vi "Find VI with Focus__ogtk.vi"(8 "error in":errorcluster caption="error in (no error)", 9 "Exclude Callers":bool=TRUE caption="Exclude All Callers (T)", 10 "Exclude Levels":i32=-1 caption="Exclude Levels (call chain=-1)", 11 "Exclude Names":string[](array[string]) caption="Exclude Names (none)") -> (0 "error out":errorcluster, 1 "Changed?":bool, 2 "VI with Focus":refnum<vi>, 3 "Valid?":bool, 5 "VI Name":string)   [LabVIEW 2017]
doc: "Returns a reference to the frontmost VI panel. \n\nThis VI is reentrant (as indicated by the crosshatched background) so that references in use by one caller aren't closed by another. This also allows different callers to exclude different panels from consideration and to get a proper indication of whether a changed has occurred since their own last last call.\n\nThis is an enhancement of Jim Kring's Find Frontmost VI that returns a reference as well as a name, signals if this has changed since the last call, allows exclusion of VIs in the calling sequence of this VI or other VIs of the user's choice (useful for editing utilities that stay on top of all other windows), cleans up unused references, and runs, on average, 50 or more times faster.\n\nGenerates no errors.\n\nCopyright © 2003 by Paul F. Sullivan. All rights reserved. You are only permitted the usage indicated in your license agreement."
uses:
  <userlib>/_OpenG.lib/appcontrol/appcontrol.llb/Find Focus State__ogtk.ctl
panel:
  out "State Data":T2={"State"=enum."Excluded?", "Recent VI"=refnum, "Recent Number"=0, "Recent VI Name"="", "VI with Focus"=refnum, "Focus Number"=0, "Focus VI Name"="", "Valid?"=FALSE, "Changed?"=FALSE} {"Focus Number" format="%.0x"; "Recent Number" format="%.0x"}
  in  "State Data":T2={"State"=enum."Recent?", "Recent VI"=refnum, "Recent Number"=0, "Recent VI Name"="", "VI with Focus"=refnum, "Focus Number"=0, "Focus VI Name"="", "Valid?"=FALSE, "Changed?"=FALSE} {"Focus Number" format="%.0x"; "Recent Number" format="%.0x"}
  # "Find VI with Focus.vi\n\nReturns a reference to the frontmost VI panel.\n\nPlease visit http://www.OpenG.org to learn about the\nOpen Source LabVIEW software movement.\n\nNOTICE -- YOU MUST LEAVE THIS NOTICE IN PLACE.  PER THE TERMS OF THE LICENSE BELOW, YOU MAY SUBLICENSE THIS SOFTWARE \nIN ANY WAY THAT DOES NOT CONFLICT WITH THIS LICENSE.\n\n### BSD License (http://www.opensource.org/licenses/bsd-license.php) Begin ###\n \nCopyright (c) 2003, Paul F. Sullivan <Paul@SULLutions.com>\n\nAll rights reserved.\n\nRedistribution and use in source and binary forms, with or without modification, are permitted provided that the following conditions are met:\n\n    * Redistributions of source code must retain the above copyright notice, this list of conditions and the following disclaimer.\n    * Redistributions in binary form must reproduce the above copyright notice, this list of conditions and the following disclaimer in the \n       documentation and/or other materials provided with the distribution.\n    * Neither the name of SciWare, James Kring, Inc., nor the names of its contributors may be used to endorse or promote products derived \n       from this software without specific prior written permission.\n\nTHIS SOFTWARE IS PROVIDED BY THE COPYRIGHT HOLDERS AND CONTRIBUTORS \"AS IS\" AND ANY EXPRESS OR IMPLIED WARRANTIES, \nINCLUDING, BUT NOT LIMITED TO, THE IMPLIED WARRANTIES OF MERCHANTABILITY AND FITNESS FOR A PARTICULAR PURPOSE ARE \nDISCLAIMED. IN NO EVENT SHALL THE COPYRIGHT OWNER OR CONTRIBUTORS BE LIABLE FOR ANY DIRECT, INDIRECT, INCIDENTAL,\n SPECIAL, EXEMPLARY, OR CONSEQUENTIAL DAMAGES (INCLUDING, BUT NOT LIMITED TO, PROCUREMENT OF SUBSTITUTE GOODS OR \nSERVICES; LOSS OF USE, DATA, OR PROFITS; OR BUSINESS INTERRUPTION) HOWEVER CAUSED AND ON ANY THEORY OF LIABILITY, \nWHETHER IN CONTRACT, STRICT LIABILITY, OR TORT (INCLUDING NEGLIGENCE OR OTHERWISE) ARISING IN ANY WAY OUT OF THE USE \nOF THIS SOFTWARE, EVEN IF ADVISED OF THE POSSIBILITY OF SUCH DAMAGE.\n\n### BSD License End ###"
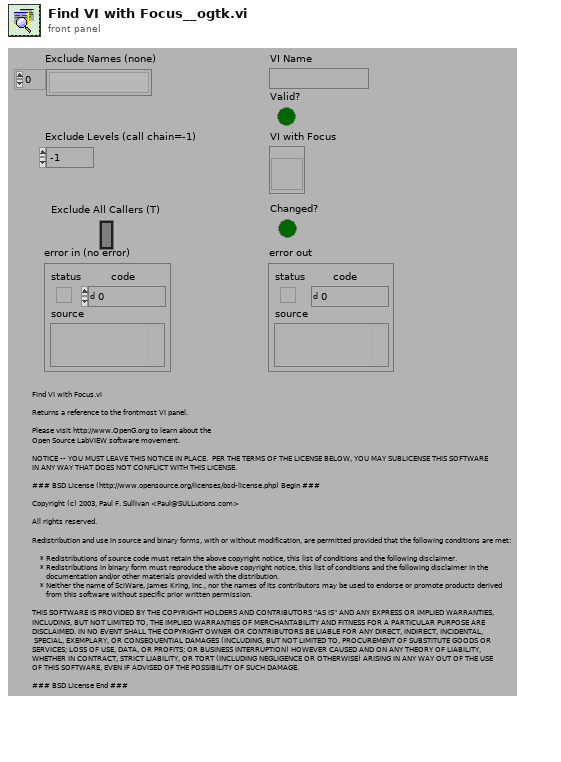
[diagram p1: front panel]
types:
  T1 = typedef "Find Focus State__ogtk.ctl" = enum16{"Initialize", "Recent?", "Accepted?", "Excluded?", "VI Panel?", "Valid?", "Done"}
  T2 = cluster{"State":T1, "Recent VI":refnum<vi>, "Recent Number":u32, "Recent VI Name":string, "VI with Focus":refnum<vi>, "Focus Number":u32, "Focus VI Name":string, "Valid?":bool, "Changed?":bool}
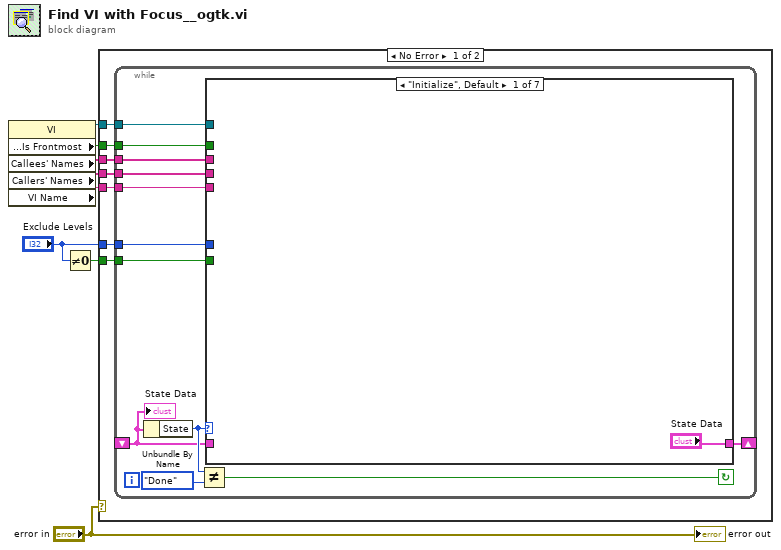
[diagram p0: block diagram]
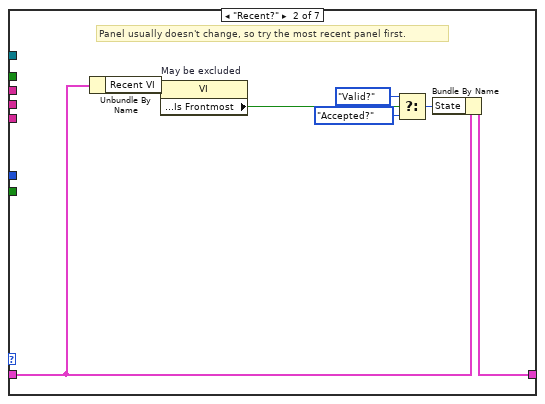
[diagram p2: hidden frame]
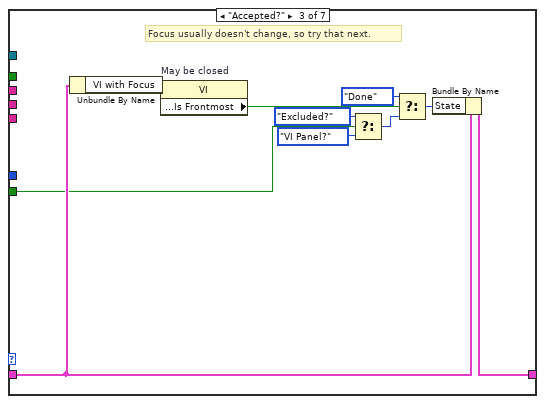
[diagram p3: hidden frame]
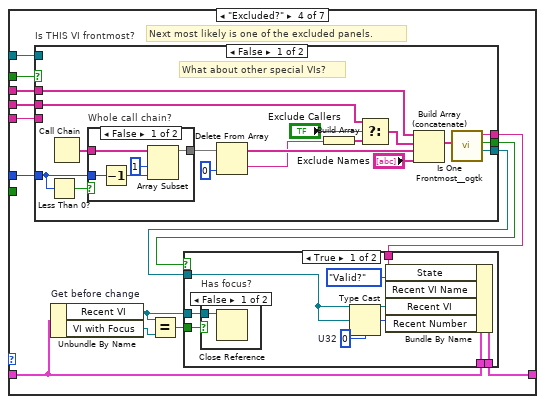
[diagram p4: hidden frame]
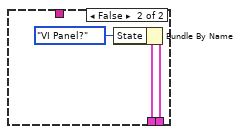
[diagram p6: hidden frame]
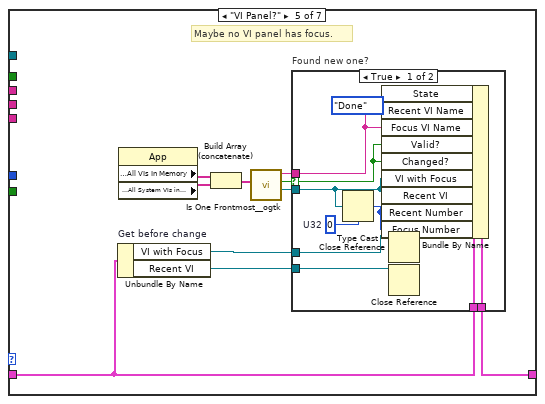
[diagram p9: hidden frame]
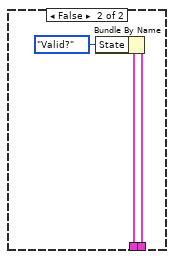
[diagram p10: hidden frame]
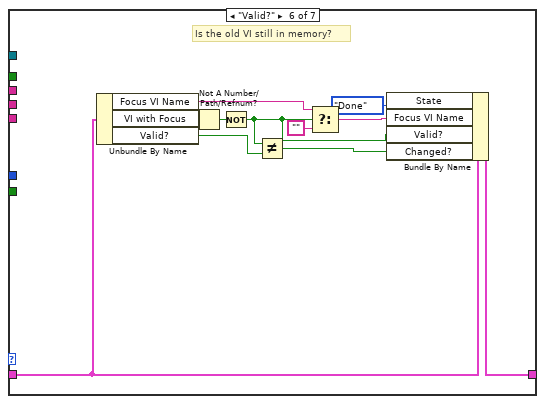
[diagram p11: hidden frame]
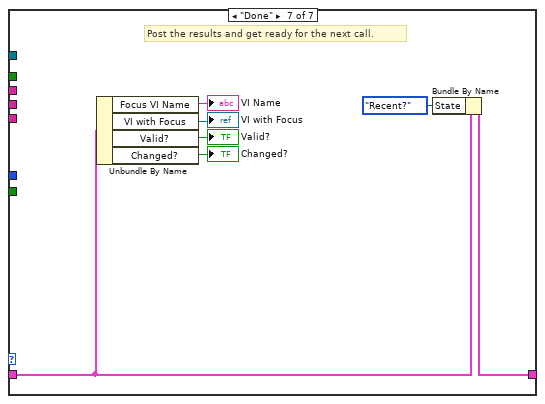
[diagram p12: hidden frame]
diagram:
  n1 = property class="VI"() -> (reference out=w4:refnum<vi>, "Front Panel Window:Is Frontmost"=w5:bool, "Callees' Names"=w7:string[], "Callers' Names"=w6:string[], "VI Name"=w1:string)  [unwired: 2 in, 1 out]
  n2 = Not Equal To 0?(x="Exclude Levels") -> (x != 0?=w2:bool)
  n3 = case shown="No Error" "error in" {
    tunnel: w6 -> [w15 _]
    tunnel: w7 -> [w14 _]
    tunnel: w5 -> [w13 _]
    tunnel: w4 -> [w12 _]
    tunnel: "Exclude Levels" -> [w11 _]
    tunnel: w2 -> [w10 _]
    tunnel: w1 -> [w9 _]
    frame No Error {
      n4 = while {
        tunnel: w9 -> [w17]
        tunnel: w10 -> [w19]
        tunnel: w11 -> [w20]
        tunnel: w12 -> [w18]
        tunnel: w13 -> [w21]
        tunnel: w14 -> [w22]
        tunnel: w15 -> [w23]
        shift-left: _ -> [w16]
        shift-right: [w25] -> _
        stop <- w24 continue-if-true
        n5 = Unbundle By Name(w16) -> ("State"=w26:T1)
        n6 = Not Equal?(x=w26, y=Find_Focus_State__ogtk."Done" ("State")) -> (x != y?=w24:bool)
        n7 = case shown="\"Initialize\", Default" w26 {
          tunnel: w21 -> [_ _ _ w59 _ _ _]
          tunnel: w23 -> [_ _ _ w58 _ _ _]
          tunnel: w22 -> [_ _ _ w57 _ _ _]
          tunnel: w20 -> [_ _ _ w56 _ _ _]
          tunnel: w19 -> [_ _ w37 _ _ _ _]
          tunnel: w16 -> [_ w34 w44 w49 w99 w129 w136]
          tunnel: ["State Data" w33 w43 w55 w104 w128 w135] -> w25
          tunnel: w18 -> [_ _ _ w52 _ _ _]
          tunnel: w17 -> [_ _ _ w50 _ _ _]
          frame "Initialize", Default {
          }
          frame "Recent?" {
            # "Panel usually doesn't change, so try the most recent panel first."
            n8 = Unbundle By Name(w34) -> ("Recent VI"=w35:refnum<vi>)
            n9 = property on="May be excluded" class="VI"(reference=w35) -> ("Front Panel Window:Is Frontmost"=w31:bool)  [unwired: 1 in, 2 out]
            n10 = Select(t=Find_Focus_State__ogtk."Valid?" ("State"), s=w31, f=Find_Focus_State__ogtk."Accepted?" ("State")) -> (s? t:f=w32:T1)
            n11 = Bundle By Name(cluster=w34, "State"=w32) -> (w33:T2)
          }
          frame "Accepted?" {
            # "Focus usually doesn't change, so try that next."
            n12 = Unbundle By Name(w44) -> ("VI with Focus"=w45:refnum<vi>)
            n13 = property on="May be closed" class="VI"(reference=w45) -> ("Front Panel Window:Is Frontmost"=w41:bool)  [unwired: 1 in, 2 out]
            n14 = Select(t=Find_Focus_State__ogtk."Excluded?" ("State"), s=w37, f=Find_Focus_State__ogtk."VI Panel?" ("State")) -> (s? t:f=w38:T1)
            n15 = Select(t=Find_Focus_State__ogtk."Done" ("State"), s=w41, f=w38) -> (s? t:f=w42:T1)
            n16 = Bundle By Name(cluster=w44, "State"=w42) -> (w43:T2)
          }
          frame "Excluded?" {
            # "Next most likely is one of the excluded panels."
            n17 = case "Is THIS VI frontmost?" shown="False" w59 {
              selector: w59 -> [_ w98]
              tunnel: w56 -> [w76 _]
              tunnel: [w75 w98] -> w54
              tunnel: w58 -> [w85 _]
              tunnel: w57 -> [w80 _]
              tunnel: [w74 w97] -> w53
              tunnel: w52 -> [_ w97]
              tunnel: [w73 w96] -> w51
              tunnel: w50 -> [_ w96]
              frame False {
                # "What about other special VIs?"
                n18 = Less Than 0?(x=w76) -> (x < 0?=w87:bool)
                n19 = Call Chain() -> (call chain=w88:string[])
                n20 = case "Whole call chain?" shown="False" w87 {
                  tunnel: w76 -> [w94 _]
                  tunnel: [w91 w95] -> w84
                  tunnel: w88 -> [w90 w95]
                  frame False {
                    n21 = Decrement(x=w94) -> (x-1=w92:i32)
                    n22 = Array Subset(array=w90, index=1 ("Array Index"), length=w92) -> (w91:string[])
                  }
                  frame True {
                  }
                }
                n23 = Delete From Array(array=w84, index=0 ("Index")) -> (deleted portion=w82:string, array with subset deleted=w86:string[])  [unwired: 1 in]
                n24 = Build Array(w82) -> (w81:string[])
                n25 = Select(t=w85, s="Exclude Callers", f=w81) -> (s? t:f=w79:string[])
                n26 = Build Array (concatenate)(w80, w79, w86, "Exclude Names") -> (w89:string[])
                n27 = call <userlib>:"Is One Frontmost__ogtk.vi"("VI names"=w89) -> ("VI Refnum"=w74:refnum<vi>, "yes"=w75:bool, "VI name"=w73:string)  [unwired: 7 in, 1 out]
              }
              frame True {
              }
            }
            n28 = Unbundle By Name "Get before change"(w49) -> ("Recent VI"=w47:refnum<vi>, "VI with Focus"=w48:refnum<vi>)
            n29 = Equal?(x=w47, y=w48) -> (x = y?=w46:bool)
            n30 = case shown="True" w54 {
              tunnel: [w68 w72] -> w55
              tunnel: w49 -> [w67 w71]
              tunnel: w53 -> [w63 _]
              tunnel: w47 -> [w65 _]
              tunnel: w51 -> [w60 _]
              tunnel: w46 -> [w61 _]
              frame True {
                w62 = u32 0  # U32
                n31 = case "Has focus?" shown="False" w61 {
                  tunnel: w65 -> [w69 _]
                  frame False {
                    n32 = Close Reference(reference=w69) -> ()  [unwired: 1 in, 1 out]
                  }
                  frame True {
                  }
                }
                n33 = Type Cast(type=w62, x=w63) -> (*(type *) &x=w64:u32)
                n34 = Bundle By Name(cluster=w67, "State"=Find_Focus_State__ogtk."Valid?", "Recent VI Name"=w60, "Recent VI"=w63, "Recent Number"=w64) -> (w68:T2)
              }
              frame False {
                n35 = Bundle By Name(cluster=w71, "State"=Find_Focus_State__ogtk."VI Panel?") -> (w72:T2)
              }
            }
          }
          frame "VI Panel?" {
            # "Maybe no VI panel has focus."
            n36 = Unbundle By Name "Get before change"(w99) -> ("VI with Focus"=w101:refnum<vi>, "Recent VI"=w100:refnum<vi>)
            n37 = property class="App"() -> ("Application:All VIs In Memory"=w108:string[], "Application:All System VIs in Memory"=w107:string[])  [unwired: 2 in, 2 out]
            n38 = Build Array (concatenate)(w108, w107) -> (w106:string[])
            n39 = call <userlib>:"Is One Frontmost__ogtk.vi"("VI names"=w106) -> ("VI Refnum"=w102:refnum<vi>, "yes"=w105:bool, "VI name"=w103:string)  [unwired: 7 in, 1 out]
            n40 = case "Found new one?" shown="True" w105 {
              selector: w105 -> [w116 _]
              tunnel: w99 -> [w118 w121]
              tunnel: [w117 w120] -> w104
              tunnel: w103 -> [w114 _]
              tunnel: w102 -> [w110 _]
              tunnel: w101 -> [w112 _]
              tunnel: w100 -> [w113 _]
              frame True {
                w111 = u32 0  # U32
                n41 = Type Cast(type=w111, x=w110) -> (*(type *) &x=w109:u32)
                n42 = Bundle By Name(cluster=w118, "State"=Find_Focus_State__ogtk."Done", "Recent VI Name"=w114, "Focus VI Name"=w114, "Valid?"=w116, "Changed?"=w116, "VI with Focus"=w110, "Recent VI"=w110, "Recent Number"=w109, "Focus Number"=w109) -> (w117:T2)
                n43 = Close Reference(reference=w112) -> ()  [unwired: 1 in, 1 out]
                n44 = Close Reference(reference=w113) -> ()  [unwired: 1 in, 1 out]
              }
              frame False {
                n45 = Bundle By Name(cluster=w121, "State"=Find_Focus_State__ogtk."Valid?") -> (w120:T2)
              }
            }
          }
          frame "Valid?" {
            # "Is the old VI still in memory?"
            n46 = Unbundle By Name(w129) -> ("Focus VI Name"=w124:string, "VI with Focus"=w132:refnum<vi>, "Valid?"=w130:bool)
            n47 = Not A Number/Path/Refnum?(number/path/refnum=w132) -> (NaN/Path/Refnum?=w131:bool)
            n48 = Not(x=w131) -> (.not. x?=w123:bool)
            n49 = Not Equal?(x=w123, y=w130) -> (x != y?=w127:bool)
            n50 = Select(t=w124, s=w123, f="") -> (s? t:f=w126:string)
            n51 = Bundle By Name(cluster=w129, "State"=Find_Focus_State__ogtk."Done", "Focus VI Name"=w126, "Valid?"=w123, "Changed?"=w127) -> (w128:T2)
          }
          frame "Done" {
            # "Post the results and get ready for the next call."
            n52 = Unbundle By Name(w136) -> ("Focus VI Name"=→"VI Name":string, "VI with Focus"=→"VI with Focus":refnum<vi>, "Valid?"=→"Valid?":bool, "Changed?"=→"Changed?":bool)
            n53 = Bundle By Name(cluster=w136, "State"=Find_Focus_State__ogtk."Recent?") -> (w135:T2)
          }
        }
        "State Data" <- w16
      }
    }
    frame Error {
    }
  }
  "error out" <- "error in"
